vi "ResolveCollisonWithOther.vi"(0 "Snake 1 X's":i32[](array[numeric])=[490, 500, 500, 500, 500, 500, 500, 500, 500, 500, 500, 500, 500, 500, 500, 500, 500, 500, 500, 500, 500, 500, 500, 500, 500, 500], 2 "Snake1X":i32=490, 4 "Snake2X":i32=640, 6 "Snake1Y":i32=500, 7 "Snake 1 Y's":i32[](array[numeric])=[500, 500, 500, 500, 500, 500, 500, 500, 500, 500, 500, 500, 500, 500, 500, 500, 500, 500, 500, 500, 500, 500, 500, 500, 500, 500], 8 "Snake 2 Y's":i32[](array[numeric])=[500, 500, 500, 500, 500, 500, 500, 500, 500, 500, 500, 500, 500, 500, 500, 500, 500, 500, 500, 500, 500, 500, 500, 500, 500, 500, 500, 500, 500, 500, 500, 500, 500, 500, 500, 500, 500], 9 "Snake 2 X's":i32[](array[numeric])=[640, 630, 620, 610, 600, 590, 580, 570, 560, 550, 540, 530, 520, 510, 500, 500, 500, 500, 500, 500, 500, 500, 500, 500, 500, 500, 500, 500, 500, 500, 500, 500, 500, 500, 500, 500, 500], 10 "Snake2Y":i32=1000) -> (18 "Snake 1 Died":bool, 19 "Snake 2 Died":bool)   [LabVIEW 2012]
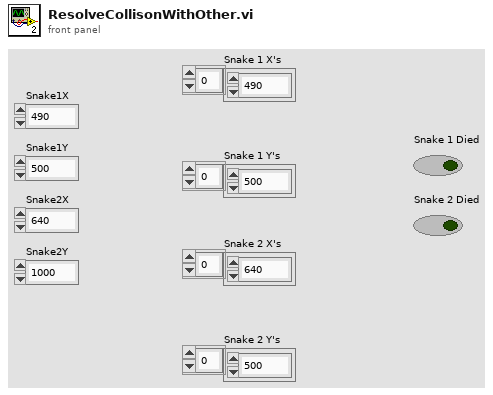
[diagram p1: front panel]
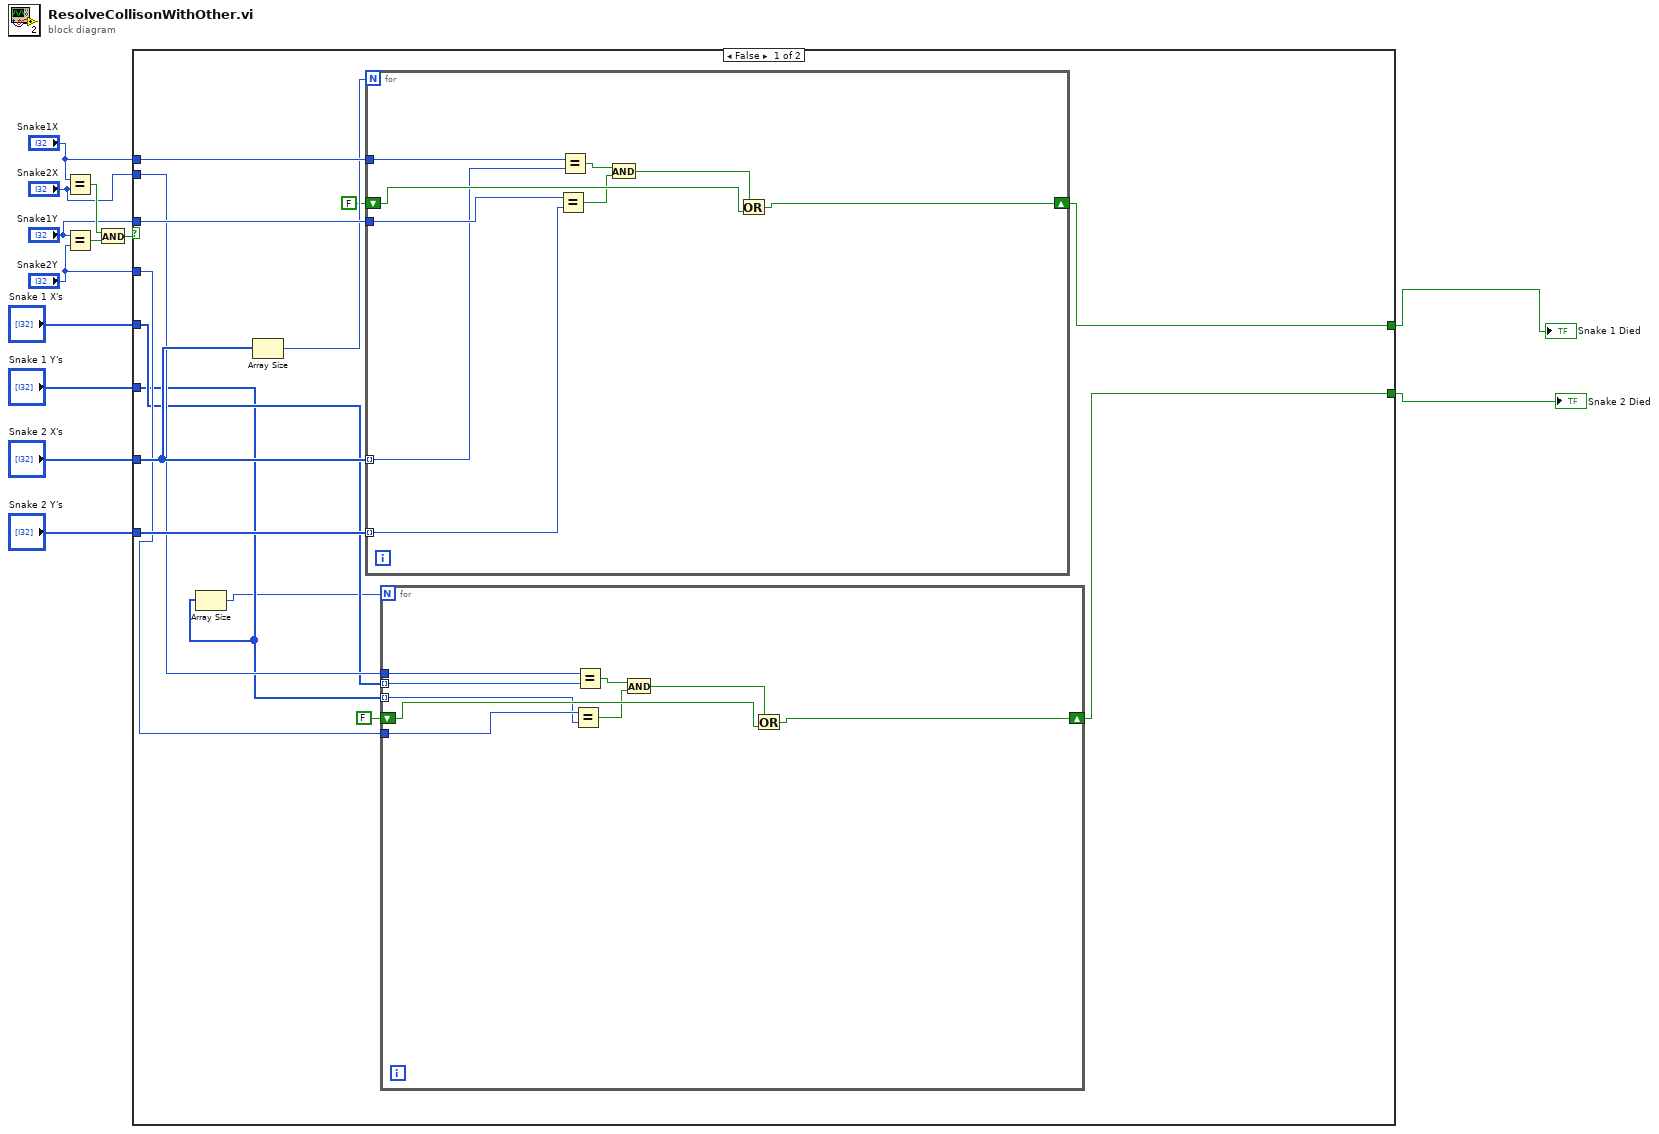
[diagram p0: block diagram]
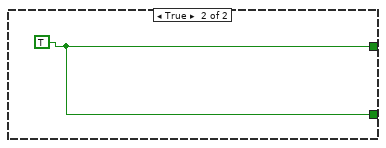
[diagram p2: hidden frame]
diagram:
  n1 = Equal?(x="Snake1X", y="Snake2X") -> (x = y?=w13:bool)
  n2 = Equal?(x="Snake1Y", y="Snake2Y") -> (x = y?=w12:bool)
  n3 = And(x=w13, y=w12) -> (x .and. y?=w11:bool)
  n4 = case shown="False" w11 {
    tunnel: "Snake 1 X's" -> [w19 _]
    tunnel: "Snake 1 Y's" -> [w18 _]
    tunnel: "Snake 2 X's" -> [w23 _]
    tunnel: "Snake 2 Y's" -> [w27 _]
    tunnel: "Snake1Y" -> [w26 _]
    tunnel: "Snake2Y" -> [w20 _]
    tunnel: "Snake1X" -> [w25 _]
    tunnel: "Snake2X" -> [w21 _]
    tunnel: [w16 w46] -> w1
    tunnel: [w24 w46] -> w2
    frame False {
      n5 = Array Size(array=w18) -> (size(s)=w17:i32)
      n6 = Array Size(array=w23) -> (size(s)=w22:i32)
      n7 = for {
        N: w22 -> [_]
        shift-right: [w39] -> w24
        shift-left: FALSE -> [w45]
        tunnel: w23 -> [w38] mode=indexing
        tunnel: w27 -> [w37] mode=indexing
        tunnel: w26 -> [w41]
        tunnel: w25 -> [w44]
        n8 = Equal?(x=w41, y=w37) -> (x = y?=w42:bool)
        n9 = Equal?(x=w44, y=w38) -> (x = y?=w43:bool)
        n10 = And(x=w43, y=w42) -> (x .and. y?=w40:bool)
        n11 = Or(x=w40, y=w45) -> (x .or. y?=w39:bool)
      }
      n12 = for {
        N: w17 -> [_]
        shift-right: [w32] -> w16
        shift-left: FALSE -> [w36]
        tunnel: w21 -> [w31]
        tunnel: w20 -> [w30]
        tunnel: w19 -> [w29] mode=indexing
        tunnel: w18 -> [w28] mode=indexing
        n13 = Equal?(x=w30, y=w28) -> (x = y?=w34:bool)
        n14 = Equal?(x=w31, y=w29) -> (x = y?=w35:bool)
        n15 = And(x=w35, y=w34) -> (x .and. y?=w33:bool)
        n16 = Or(x=w33, y=w36) -> (x .or. y?=w32:bool)
      }
    }
    frame True {
      w46 = TRUE
    }
  }
  "Snake 1 Died" <- w2
  "Snake 2 Died" <- w1
